vi "LSMcontroller_v58.vi"() -> ()   [LabVIEW 2015] (continued)
                n2596 = call <vilib>:"DAQmx Start Task.vi"("task/channels in"=w5606, "error in"=w5607) -> ("task out"=w5608:refnum<k21>, "error out"=w5609:errorcluster)  [unwired: 12 in]
                n2597 = call <vilib>:"DAQmx Stop Task.vi"("task/channels in"=w5608, "error in"=w5609) -> ("task out"=w5610:refnum<k21>, "error out"=w5611:errorcluster)  [unwired: 12 in]
                n2598 = call <vilib>:"DAQmx Clear Task.vi"("task in"=w5610, "error in"=w5611) -> ()  [unwired: 13 in, 1 out]
              }
            }
          }
          event "sealtest": Value Change {
            n2599 = event-data() -> ()  [unwired: 1 in, 6 out]
            n2600 = case shown="True" "sealtest" {
              frame False {
              }
              frame True {
                n2601 = stacked-sequence {
                  seq-local: [w5613 _ _ _ _ _] -> [_ w5646 _ w5698 _ _]
                  frame #0 {
                    n2602 = stacked-sequence {
                      tunnel: [_ w5625 _] -> w5613
                      frame #0 {
                        n2603 = call "2pparameters.vi"("command"="get") -> ("params out"=w5618:T12)  [unwired: 1 in]
                        n2604 = Unbundle By Name(w5618) -> ("autoshutter"=w5619:bool)
                        n2605 = local read "OCchecked?"() -> (w5616:bool)
                        n2606 = call "sealtestwfparams.vi"("command"="set") -> ()  [unwired: 6 in, 1 out]
                        n2607 = case shown="False" w5616 {
                          frame False {
                            n2608 = One Button Dialog(message="Is the OC gain correct?", button name ("OK")="ok") -> (true=w5620:bool)
                            n2609 = local write "OCchecked?"(w5620) -> ()
                          }
                          frame True {
                          }
                        }
                        n2610 = case shown="True" w5619 {
                          frame False {
                          }
                          frame True {
                            n2611 = call "shuttercontrol.vi"("command"="close") -> ()  [unwired: 1 in, 1 out]
                          }
                        }
                        n2612 = call "allAI-temp.vi"("command"=enum16{"get", "set", "clear", "append"}."clear") -> ()  [unwired: 3 in, 2 out]
                      }
                      frame #1 {
                        n2613 = call "sealtestwfparams.vi"("command"="get") -> ("Params out"=w5631:T25)  [unwired: 6 in]
                        n2614 = Unbundle By Name(w5631) -> ("AO parameters"=w5629:T1)
                        "AO parameters 2" <- w5629
                        n2615 = Index Array(array=w5629, index=0) -> (element=w5628:T26)
                        n2616 = call "generateRampedSquareWave_fromAOparameters.vi"("AO params"=w5628) -> ("Waveform"=w5624:waveform(dbl), "wflength"=w5625:i32)
                        "Waveform Graph" <- w5624
                        "wflength" <- w5625
                        n2617 = Build Array(w5624) -> (w5627:waveform(dbl)[])
                        n2618 = call "waveformssealtestbuffer.vi"("AO wf in"=w5627, "command"="set") -> ()  [unwired: 1 out]
                      }
                      frame #2 {
                        n2619 = local read "Vholding (mV)"() -> (w5634:sgl)
                        n2620 = local read "Current Clamp"() -> (w5640:bool)
                        n2621 = local read "Voltage Clamp"() -> (w5639:bool)
                        n2622 = local read "OCgain"() -> (w5635:sgl)
                        n2623 = local read "CC_ICgain"() -> (w5638:dbl)
                        n2624 = local read "holdon"() -> (w5633:bool)
                        n2625 = call "patchparameters.vi"("command"="get") -> ("Params out"=w5642:T15)  [unwired: 1 in]
                        n2626 = Bundle By Name(cluster=w5642, "VC"=w5639, "CC"=w5640, "CC_icg (pA/mv)"=w5638, "VC_icg (mV/mV)"=10.0, "OCG (mV/pA)"=w5635, "OVG (mV/mV)"=0.1, "Vhold (mV)"=w5634, "holdon"=w5633) -> (w5641:T15)
                        n2627 = call "patchparameters.vi"("Params in"=w5641, "command"="set") -> ()  [unwired: 1 out]
                      }
                    }
                  }
                  frame #1 {
                    w5645 = 2
                    n2628 = call "patchparameters.vi"("command"="get") -> ("Params out"=w5653:T15)  [unwired: 1 in]
                    n2629 = Unbundle By Name(w5653) -> ("holdon"=w5652:bool, "Vhold (mV)"=w5651:sgl, "CC_icg (pA/mv)"=w5659:sgl, "CC"=w5657:bool, "VC_icg (mV/mV)"=w5658:sgl)
                    n2630 = Select(t=w5659, s=w5657, f=w5658) -> (s? t:f=w5660:sgl)
                    n2631 = To Single Precision Float(number=0.001 ("y")) -> (single precision float=w5661:sgl)
                    n2632 = Compound Arithmetic op=MULTIPLY(w5651, w5660, w5661) -> (w5655:sgl)
                    n2633 = case shown="False" w5652 {
                      tunnel: w5655 -> [_ w5673]
                      tunnel: [0.0 w5673] -> w5648
                      frame False {
                      }
                      frame True {
                      }
                    }
                    n2634 = Greater Than 0?(x=w5645) -> (x > 0?=w5647:bool)
                    n2635 = case shown="True" w5647 {
                      tunnel: w5646 -> [_ w5662]
                      tunnel: w5645 -> [_ w5665]
                      frame False {
                      }
                      frame True {
                        n2636 = Initialize Array(sgl 0.0 ("element"), w5665, w5662) -> (w5663:sgl[][])
                        n2637 = call "allAI-temp.vi"("array in"=w5663, "command"=enum16{"get", "set", "clear", "append"}."set") -> ()  [unwired: 2 in, 2 out]
                      }
                    }
                    n2638 = flat-sequence {
                      tunnel: w5646 -> [w5669]
                      tunnel: w5646 -> [w5668]
                      tunnel: [w5668] -> w5650
                      tunnel: [w5667] -> w5649
                      tunnel: w5648 -> [w5667]
                      tunnel: w5650 -> [w5671]
                      tunnel: w5649 -> [w5670]
                      frame #0 {
                        n2639 = call "prepAI_sealtest.vi"("samples per channel"=w5669) -> ()  [unwired: 2 in]
                      }
                      frame #1 {
                        n2640 = call "prepAO_sealtest.vi"("Vhold"=w5670, "samples per channel"=w5671) -> ()  [unwired: 1 in]
                      }
                    }
                  }
                  frame #2 {
                    n2641 = stacked-sequence {
                      frame #0 {
                        n2642 = call "tempconfigAO.vi"("command"="get") -> ("Temp Config out"=w5677:T27)  [unwired: 1 in]
                        n2643 = Unbundle By Name(w5677) -> ("AO"=w5678:refnum<k21>[], "E_AO"=w5679:errorcluster[])
                        n2644 = for {
                          tunnel: w5678 -> [w5687] mode=indexing
                          tunnel: w5679 -> [w5686] mode=indexing
                          tunnel: [w5685] -> w5681 mode=indexing
                          tunnel: [w5684] -> w5682 mode=indexing
                          n2645 = call <vilib>:"DAQmx Start Task.vi"("task/channels in"=w5687, "error in"=w5686) -> ("task out"=w5685:refnum<k21>, "error out"=w5684:errorcluster)  [unwired: 12 in]
                        }
                        n2646 = call "tempconfigAO.vi"("command"="get") -> ("Temp Config out"=w5680:T27)  [unwired: 1 in]
                        n2647 = Bundle By Name(cluster=w5680, "AO"=w5681, "E_AO"=w5682) -> (w5683:T27)
                        n2648 = call "tempconfigAO.vi"("Temp Config in"=w5683, "command"="set") -> ()  [unwired: 1 out]
                      }
                      frame #1 {
                        n2649 = call "tempconfigAI.vi"("command"="get") -> ("Temp Config out"=w5689:T28)  [unwired: 1 in]
                        n2650 = Unbundle By Name(w5689) -> ("AI"=w5694:refnum<k21>, "E_AI"=w5695:errorcluster)
                        n2651 = call <vilib>:"DAQmx Start Task.vi"("task/channels in"=w5694, "error in"=w5695) -> ("task out"=w5696:refnum<k21>, "error out"=w5697:errorcluster)  [unwired: 12 in]
                        n2652 = call "tempconfigAI.vi"("command"="get") -> ("Temp Config out"=w5691:T28)  [unwired: 1 in]
                        n2653 = Bundle By Name(cluster=w5691, "AI"=w5696, "E_AI"=w5697) -> (w5693:T28)
                        n2654 = call "tempconfigAI.vi"("Temp Config in"=w5693, "command"="set") -> ()  [unwired: 1 out]
                      }
                    }
                  }
                  frame #3 {
                    n2655 = while {
                      tunnel: w5698 -> [w5699]
                      stop <- w5700 stop-if-true
                      n2656 = local read "sealtest"() -> (w5703:bool)
                      n2657 = Not(x=w5703) -> (.not. x?=w5702:bool)
                      n2658 = case shown="False" w5702 {
                        tunnel: w5699 -> [w5704 _]
                        frame False {
                          n2659 = stacked-sequence {
                            seq-local: [_ _ _ w5743 _ _] -> [_ _ _ _ w5799 _]
                            seq-local: [w5705 _ _ _ _ _] -> [_ w5714 _ w5736 w5788 w5819]
                            tunnel: w5704 -> [_ _ w5722 _ w5787 _]
                            frame #0 {
                              n2660 = call "patchparameters.vi"("command"="get") -> ("Params out"=w5712:T15)  [unwired: 1 in]
                              n2661 = local read "Vholding (mV)"() -> (w5709:sgl)
                              n2662 = Unbundle By Name(w5712) -> ("Vhold (mV)"=w5708:sgl, "holdon"=w5711:bool)
                              n2663 = local read "holdon"() -> (w5710:bool)
                              n2664 = Not Equal?(x=w5709, y=w5708) -> (x != y?=w5707:bool)
                              n2665 = Not Equal?(x=w5711, y=w5710) -> (x != y?=w5706:bool)
                              n2666 = Or(x=w5707, y=w5706) -> (x .or. y?=w5705:bool)
                            }
                            frame #1 {
                              n2667 = case shown="True" w5714 {
                                frame False {
                                }
                                frame True {
                                n2668 = local read "Vholding (mV)"() -> (w5717:sgl)
                                n2669 = local read "holdon"() -> (w5715:bool)
                                n2670 = call "patchparameters.vi"("command"="get") -> ("Params out"=w5718:T15)  [unwired: 1 in]
                                n2671 = Bundle By Name(cluster=w5718, "Vhold (mV)"=w5717, "holdon"=w5715) -> (w5716:T15)
                                n2672 = call "patchparameters.vi"("Params in"=w5716, "command"="set") -> ()  [unwired: 1 out]
                                }
                              }
                            }
                            frame #2 {
                              n2673 = call "tempconfigAI.vi"("command"="get") -> ("Temp Config out"=w5732:T28)  [unwired: 1 in]
                              n2674 = Unbundle By Name(w5732) -> ("AI"=w5731:refnum<k21>, "E_AI"=w5730:errorcluster)
                              n2675 = call-poly <vilib>:"DAQmx Read.vi"("task/channels in"=w5731, "number of samples per channel"=w5722, "timeout"=10.0, "error in"=w5730) -> ("task out"=w5726:refnum<k21>, "data"=w5723:i16[][], "error out"=w5735:errorcluster)  [unwired: 9 in]
                              n2676 = call "tempconfigAI.vi"("command"="get") -> ("Temp Config out"=w5727:T28)  [unwired: 1 in]
                              n2677 = Bundle By Name(cluster=w5727, "AI"=w5726, "E_AI"=w5735) -> (w5734:T28)
                              n2678 = To Single Precision Float(number=w5723) -> (single precision float=w5725:sgl[][])
                              n2679 = call "tempconfigAI.vi"("Temp Config in"=w5734, "command"="set") -> ()  [unwired: 1 out]
                              n2680 = call "allAI-temp.vi"("array in"=w5725, "command"=enum16{"get", "set", "clear", "append"}."set") -> ()  [unwired: 2 in, 2 out]
                            }
                            frame #3 {
                              n2681 = case shown="True" w5736 {
                                frame False {
                                }
                                frame True {
                                n2682 = call "tempconfigAO.vi"("command"="get") -> ("Temp Config out"=w5776:T27)  [unwired: 1 in]
                                n2683 = Unbundle By Name(w5776) -> ("AO"=w5775:refnum<k21>[], "E_AO"=w5774:errorcluster[])
                                n2684 = call "tempconfigAI.vi"("command"="get") -> ("Temp Config out"=w5763:T28)  [unwired: 1 in]
                                n2685 = Unbundle By Name(w5763) -> ("AI"=w5764:refnum<k21>, "E_AI"=w5765:errorcluster)
                                n2686 = for {
                                tunnel: w5775 -> [w5780] mode=indexing
                                tunnel: w5774 -> [w5779] mode=indexing
                                tunnel: [w5778] -> w5770 mode=indexing
                                n2687 = call <vilib>:"DAQmx Stop Task.vi"("task/channels in"=w5780, "error in"=w5779) -> ("task out"=w5781:refnum<k21>, "error out"=w5782:errorcluster)  [unwired: 12 in]
                                n2688 = call <vilib>:"DAQmx Clear Task.vi"("task in"=w5781, "error in"=w5782) -> ("error out"=w5778:errorcluster)  [unwired: 13 in]
                                }
                                n2689 = call <vilib>:"DAQmx Stop Task.vi"("task/channels in"=w5764, "error in"=w5765) -> ("task out"=w5761:refnum<k21>, "error out"=w5760:errorcluster)  [unwired: 12 in]
                                n2690 = call <vilib>:"DAQmx Clear Task.vi"("task in"=w5761, "error in"=w5760) -> ("error out"=w5759:errorcluster)  [unwired: 13 in]
                                n2691 = call "tempconfigAO.vi"("command"="get") -> ("Temp Config out"=w5771:T27)  [unwired: 1 in]
                                n2692 = Bundle By Name(cluster=w5771, "E_AO"=w5770) -> (w5769:T27)
                                n2693 = call "tempconfigAI.vi"("command"="get") -> ("Temp Config out"=w5767:T28)  [unwired: 1 in]
                                n2694 = Bundle By Name(cluster=w5767, "E_AI"=w5759) -> (w5758:T28)
                                n2695 = call "tempconfigAO.vi"("Temp Config in"=w5769, "command"="set") -> ()  [unwired: 1 out]
                                n2696 = call "tempconfigAI.vi"("Temp Config in"=w5758, "command"="set") -> ()  [unwired: 1 out]
                                }
                              }
                              n2697 = call "allAI-temp.vi"("command"=enum16{"get", "set", "clear", "append"}."get") -> ("array out"=w5740:sgl[][])  [unwired: 3 in, 1 out]
                              n2698 = call "tempconfigAI.vi"("command"="get") -> ("Temp Config out"=w5753:T28)  [unwired: 1 in]
                              n2699 = call "tempconfigAI.vi"("command"="get") -> ("Temp Config out"=w5755:T28)  [unwired: 1 in]
                              n2700 = Unbundle By Name(w5753) -> ("header"=w5751:dbl[])
                              n2701 = Unbundle By Name(w5755) -> ("header"=w5757:dbl[])
                              n2702 = Index Array(array=w5740, index (row) #1=1 ("index (row)"), index (row) #2=0 ("index (row)")) -> (element #1=w5738:sgl[], element #2=w5737:sgl[])  [unwired: 2 in]
                              n2703 = local read "OCgain"() -> (w5745:sgl)
                              n2704 = call "Unscaledtoscaled.vi"("Unscaled Data"=w5738, "Header Information"=w5751) -> ("Array"=w5750:sgl[])  [unwired: 1 in]
                              n2705 = call "Unscaledtoscaled.vi"("Unscaled Data"=w5737, "Header Information"=w5757) -> ("Array"=w5754:sgl[])  [unwired: 1 in]
                              n2706 = Multiply(x=w5750, y=0.1) -> (x*y=w5747:dbl[])
                              n2707 = Divide(x=w5754, y=w5745) -> (x/y=w5746:sgl[])
                              n2708 = Build Array(w5747, w5746) -> (w5749:dbl[][])
                              n2709 = Multiply(x=w5749, y=1000.0) -> (x*y=w5743:dbl[][])
                              "Patch readout" <- w5743
                            }
                            frame #4 {
                              n2710 = case shown="True" w5788 {
                                tunnel: w5787 -> [_ w5800]
                                frame False {
                                }
                                frame True {
                                n2711 = call "patchparameters.vi"("command"="get") -> ("Params out"=w5804:T15)  [unwired: 1 in]
                                n2712 = Unbundle By Name(w5804) -> ("holdon"=w5803:bool, "Vhold (mV)"=w5802:sgl, "CC_icg (pA/mv)"=w5810:sgl, "CC"=w5808:bool, "VC_icg (mV/mV)"=w5809:sgl)
                                n2713 = Select(t=w5810, s=w5808, f=w5809) -> (s? t:f=w5811:sgl)
                                n2714 = To Single Precision Float(number=0.001 ("y")) -> (single precision float=w5812:sgl)
                                n2715 = Compound Arithmetic op=MULTIPLY(w5802, w5811, w5812) -> (w5806:sgl)
                                n2716 = case shown="True" w5803 {
                                tunnel: w5806 -> [_ w5817]
                                tunnel: [0.0 w5817] -> w5801
                                frame False {
                                }
                                frame True {
                                }
                                }
                                n2717 = flat-sequence {
                                tunnel: w5800 -> [w5813]
                                tunnel: w5801 -> [w5815]
                                tunnel: w5800 -> [w5814]
                                frame #0 {
                                n2718 = call "prepAI_sealtest.vi"("samples per channel"=w5813) -> ()  [unwired: 2 in]
                                }
                                frame #1 {
                                n2719 = call "prepAO_sealtest.vi"("Vhold"=w5815, "samples per channel"=w5814) -> ()  [unwired: 1 in]
                                }
                                }
                                }
                              }
                              n2720 = call "sealtestwfparams.vi"("command"="get") -> ("Params out"=w5793:T25)  [unwired: 6 in]
                              n2721 = Unbundle By Name(w5793) -> ("AO parameters"=w5794:T1)
                              n2722 = Index Array(array=w5794, index=0) -> (element=w5796:T26)
                              n2723 = Unbundle By Name(w5796) -> ("Cycles"=w5791:dbl, "Start amplitude (V)"=w5790:dbl, "Sampling frequency (Hz)"=w5789:dbl)
                              n2724 = local read "fitpoints"() -> (w5797:dbl)
                              n2725 = script code="V=data(1,:);\nI=data(2,:);\ntres=mean(V);\nspc=(nsamp./ncyc);\nV=V(spc+1:end-spc);\nI=I(spc+1:end-spc);\ndV=mean(V(V>tres))-mean(V(V<tres))\nIcyc=reshape(I,[spc ncyc-2]);\nIcyc=Icyc';\nIcyc=mean(Icyc,1);\ndIss=mean(Icyc(floor(spc*0.15):floor(spc/2)-2))-mean(Icyc(spc*0.65:spc-2))\nRm=dV*1e3/dIss;\n[maxi,ind]=max(Icyc);\nIfit=Icyc(ind+1:ind+1+points-1)-0.5*(mean(Icyc(floor(spc*0.15):floor(spc/2)-2))+mean(Icyc(spc*0.65:spc-2)))\nt=(3:points-1+3)./srate*1000;\nt=t';\nIfit=Ifit';\nc=fit(t,Ifit, 'exp1');\ncoeffs=coeffvalues(c);\nIa=coeffs(1);\nRa=dV*1e3./Ia/2;\ntau=-1./coeffs(2);\ncap=tau/Ra*1000;"("data"=w5799, "nsamp"=w5787, "ncyc"=w5791, "maxV"=w5790, "points"=w5797, "srate"=w5789) -> ("cap"=w5786:dbl, "Ra"=w5785:dbl, "Icyc"=w5784:dbl[], "Rm"=w5783:dbl)  [unwired: 1 in, 1 out]
                              n2726 = local read "set as Rp?"() -> (w5798:bool)
                              n2727 = local write "Cmembrane"(w5786) -> ()
                              n2728 = local write "Rmembrane (MOhm)"(w5783) -> ()
                              n2729 = local write "Racces (MOhm)"(w5785) -> ()
                              n2730 = case shown="True" w5798 {
                                tunnel: w5783 -> [_ w5818]
                                frame False {
                                }
                                frame True {
                                n2731 = local write "Rpipette (MOhm)"(w5818) -> ()
                                }
                              }
                              n2732 = local write "Ifit"(w5784) -> ()
                            }
                            frame #5 {
                              n2733 = local read "set as Rp?"() -> (w5820:bool)
                              n2734 = case shown="True" w5819 {
                                frame False {
                                }
                                frame True {
                                n2735 = stacked-sequence {
                                frame #0 {
                                n2736 = call "tempconfigAO.vi"("command"="get") -> ("Temp Config out"=w5827:T27)  [unwired: 1 in]
                                n2737 = Unbundle By Name(w5827) -> ("AO"=w5826:refnum<k21>[], "E_AO"=w5825:errorcluster[])
                                n2738 = for {
                                tunnel: w5826 -> [w5834] mode=indexing
                                tunnel: w5825 -> [w5833] mode=indexing
                                tunnel: [w5832] -> w5823 mode=indexing
                                tunnel: [w5831] -> w5822 mode=indexing
                                n2739 = call <vilib>:"DAQmx Start Task.vi"("task/channels in"=w5834, "error in"=w5833) -> ("task out"=w5832:refnum<k21>, "error out"=w5831:errorcluster)  [unwired: 12 in]
                                }
                                n2740 = call "tempconfigAO.vi"("command"="get") -> ("Temp Config out"=w5824:T27)  [unwired: 1 in]
                                n2741 = Bundle By Name(cluster=w5824, "AO"=w5823, "E_AO"=w5822) -> (w5821:T27)
                                n2742 = call "tempconfigAO.vi"("Temp Config in"=w5821, "command"="set") -> ()  [unwired: 1 out]
                                }
                                frame #1 {
                                n2743 = call "tempconfigAI.vi"("command"="get") -> ("Temp Config out"=w5836:T28)  [unwired: 1 in]
                                n2744 = Unbundle By Name(w5836) -> ("AI"=w5841:refnum<k21>, "E_AI"=w5842:errorcluster)
                                n2745 = call <vilib>:"DAQmx Start Task.vi"("task/channels in"=w5841, "error in"=w5842) -> ("task out"=w5843:refnum<k21>, "error out"=w5844:errorcluster)  [unwired: 12 in]
                                n2746 = call "tempconfigAI.vi"("command"="get") -> ("Temp Config out"=w5838:T28)  [unwired: 1 in]
                                n2747 = Bundle By Name(cluster=w5838, "AI"=w5843, "E_AI"=w5844) -> (w5840:T28)
                                n2748 = call "tempconfigAI.vi"("Temp Config in"=w5840, "command"="set") -> ()  [unwired: 1 out]
                                }
                                }
                                }
                              }
                              n2749 = case shown="True" w5820 {
                                frame False {
                                }
                                frame True {
                                n2750 = local write "set as Rp?"(FALSE ("set as Rp?")) -> ()
                                }
                              }
                            }
                          }
                        }
                        frame True {
                        }
                      }
                      n2751 = local read "sealtest"() -> (w5701:bool)
                      n2752 = Not(x=w5701) -> (.not. x?=w5700:bool)
                    }
                  }
                  frame #4 {
                    n2753 = call "tempconfigAO.vi"("command"="get") -> ("Temp Config out"=w5871:T27)  [unwired: 1 in]
                    n2754 = Unbundle By Name(w5871) -> ("AO"=w5870:refnum<k21>[], "E_AO"=w5869:errorcluster[])
                    n2755 = call "configuration.vi"("command"="get") -> ("config out"=w5852:T13)  [unwired: 2 in, 1 out]
                    n2756 = call "tempconfigAI.vi"("command"="get") -> ("Temp Config out"=w5858:T28)  [unwired: 1 in]
                    n2757 = Unbundle By Name(w5852) -> ("Device 1 sampleclock out"=w5849:tag, "Device 1 Starttrigger out"=w5848:tag)
                    n2758 = Unbundle By Name(w5858) -> ("AI"=w5859:refnum<k21>, "E_AI"=w5860:errorcluster)
                    n2759 = for {
                      tunnel: w5870 -> [w5875] mode=indexing
                      tunnel: w5869 -> [w5874] mode=indexing
                      tunnel: [w5873] -> w5865 mode=indexing
                      n2760 = call <vilib>:"DAQmx Stop Task.vi"("task/channels in"=w5875, "error in"=w5874) -> ("task out"=w5876:refnum<k21>, "error out"=w5877:errorcluster)  [unwired: 12 in]
                      n2761 = call <vilib>:"DAQmx Clear Task.vi"("task in"=w5876, "error in"=w5877) -> ("error out"=w5873:errorcluster)  [unwired: 13 in]
                    }
                    n2762 = call <vilib>:"DAQmx Stop Task.vi"("task/channels in"=w5859, "error in"=w5860) -> ("task out"=w5856:refnum<k21>, "error out"=w5855:errorcluster)  [unwired: 12 in]
                    n2763 = call <vilib>:"DAQmx Disconnect Terminals.vi"("source terminal"=tag "/Dev1/ai/SampleClock", "destination terminal"=w5849) -> ("error out"=w5846:errorcluster)  [unwired: 13 in]
                    n2764 = call <vilib>:"DAQmx Clear Task.vi"("task in"=w5856, "error in"=w5855) -> ("error out"=w5854:errorcluster)  [unwired: 13 in]
                    n2765 = call "tempconfigAO.vi"("command"="get") -> ("Temp Config out"=w5866:T27)  [unwired: 1 in]
                    n2766 = Bundle By Name(cluster=w5866, "E_AO"=w5865) -> (w5864:T27)
                    n2767 = call "tempconfigAI.vi"("command"="get") -> ("Temp Config out"=w5862:T28)  [unwired: 1 in]
                    n2768 = Bundle By Name(cluster=w5862, "E_AI"=w5854) -> (w5853:T28)
                    n2769 = call "tempconfigAO.vi"("Temp Config in"=w5864, "command"="set") -> ()  [unwired: 1 out]
                    n2770 = call <vilib>:"DAQmx Disconnect Terminals.vi"("source terminal"=tag "/Dev1/ai/StartTrigger", "destination terminal"=w5848, "error in"=w5846) -> ()  [unwired: 12 in, 1 out]
                    n2771 = call "tempconfigAI.vi"("Temp Config in"=w5853, "command"="set") -> ()  [unwired: 1 out]
                  }
                  frame #5 {
                    w5880 = T23 4 items=["no dialog", "OK message", "continue or stop message", "OK message + warnings", "continue/stop + warnings"] ("type of dialog (OK msg:1)")
                    n2772 = call "displayerrors.vi"() -> ("error IO"=w5879:errorcluster)
                    n2773 = call "zeropatch.vi"() -> ()  [unwired: 12 in]
                    n2774 = call <vilib>:"Simple Error Handler.vi"("type of dialog (OK msg:1)"=w5880, "error in (no error)"=w5879) -> ("error out"=w5878:errorcluster)  [unwired: 3 in, 4 out]
                    n2775 = call <vilib>:"Clear Errors.vi"("error in (no error)"=w5878) -> ()  [unwired: 5 in, 2 out]
                  }
                }
              }
            }
          }
          event "readpatch": Value Change {
            n2776 = event-data() -> ()  [unwired: 1 in, 6 out]
            n2777 = local read "readpatch"() -> (w5881:bool)
            n2778 = case shown="True" w5881 {
              frame False {
              }
              frame True {
                n2779 = stacked-sequence {
                  seq-local: [w5882 _ _ _ _ _] -> [_ w5915 _ w5967 _ _]
                  frame #0 {
                    n2780 = stacked-sequence {
                      tunnel: [_ w5894 _] -> w5882
                      frame #0 {
                        n2781 = call "2pparameters.vi"("command"="get") -> ("params out"=w5887:T12)  [unwired: 1 in]
                        n2782 = Unbundle By Name(w5887) -> ("autoshutter"=w5888:bool)
                        n2783 = local read "OCchecked?"() -> (w5885:bool)
                        n2784 = call "sealtestwfparams.vi"("command"="set") -> ()  [unwired: 6 in, 1 out]
                        n2785 = case shown="False" w5885 {
                          frame False {
                            n2786 = One Button Dialog(message="Is the OC gain correct?", button name ("OK")="ok") -> (true=w5889:bool)
                            n2787 = local write "OCchecked?"(w5889) -> ()
                          }
                          frame True {
                          }
                        }
                        n2788 = case shown="True" w5888 {
                          frame False {
                          }
                          frame True {
                            n2789 = call "shuttercontrol.vi"("command"="close") -> ()  [unwired: 1 in, 1 out]
                          }
                        }
                        n2790 = call "allAI-temp.vi"("command"=enum16{"get", "set", "clear", "append"}."clear") -> ()  [unwired: 3 in, 2 out]
                      }
                      frame #1 {
                        n2791 = call "sealtestwfparams.vi"("command"="get") -> ("Params out"=w5900:T25)  [unwired: 6 in]
                        n2792 = Unbundle By Name(w5900) -> ("AO parameters"=w5898:T1)
                        n2793 = Index Array(array=w5898, index=1) -> (element=w5897:T26)
                        n2794 = call "generateRampedSquareWave_fromAOparameters.vi"("AO params"=w5897) -> ("Waveform"=w5893:waveform(dbl), "wflength"=w5894:i32)
                        n2795 = Build Array(w5893) -> (w5896:waveform(dbl)[])
                        n2796 = call "waveformssealtestbuffer.vi"("AO wf in"=w5896, "command"="set") -> ()  [unwired: 1 out]
                      }
                      frame #2 {
                        n2797 = local read "Vholding (mV)"() -> (w5903:sgl)
                        n2798 = local read "Current Clamp"() -> (w5909:bool)
                        n2799 = local read "Voltage Clamp"() -> (w5908:bool)
                        n2800 = local read "OCgain"() -> (w5904:sgl)
                        n2801 = local read "CC_ICgain"() -> (w5907:dbl)
                        n2802 = local read "holdon"() -> (w5902:bool)
                        n2803 = call "patchparameters.vi"("command"="get") -> ("Params out"=w5911:T15)  [unwired: 1 in]
                        n2804 = Bundle By Name(cluster=w5911, "VC"=w5908, "CC"=w5909, "CC_icg (pA/mv)"=w5907, "VC_icg (mV/mV)"=10.0, "OCG (mV/pA)"=w5904, "OVG (mV/mV)"=0.1, "Vhold (mV)"=w5903, "holdon"=w5902) -> (w5910:T15)
                        n2805 = call "patchparameters.vi"("Params in"=w5910, "command"="set") -> ()  [unwired: 1 out]
                      }
                    }
                  }
                  frame #1 {
                    w5914 = 2
                    n2806 = call "patchparameters.vi"("command"="get") -> ("Params out"=w5922:T15)  [unwired: 1 in]
                    n2807 = Unbundle By Name(w5922) -> ("holdon"=w5921:bool, "Vhold (mV)"=w5920:sgl, "CC_icg (pA/mv)"=w5928:sgl, "CC"=w5926:bool, "VC_icg (mV/mV)"=w5927:sgl)
                    n2808 = Select(t=w5928, s=w5926, f=w5927) -> (s? t:f=w5929:sgl)
                    n2809 = To Single Precision Float(number=0.001 ("y")) -> (single precision float=w5930:sgl)
                    n2810 = Compound Arithmetic op=MULTIPLY(w5920, w5929, w5930) -> (w5924:sgl)
                    n2811 = case shown="False" w5921 {
                      tunnel: w5924 -> [_ w5942]
                      tunnel: [0.0 w5942] -> w5917
                      frame False {
                      }
                      frame True {
                      }
                    }
                    n2812 = Greater Than 0?(x=w5914) -> (x > 0?=w5916:bool)
                    n2813 = case shown="True" w5916 {
                      tunnel: w5915 -> [_ w5931]
                      tunnel: w5914 -> [_ w5934]
                      frame False {
                      }
                      frame True {
                        n2814 = Initialize Array(sgl 0.0 ("element"), w5934, w5931) -> (w5932:sgl[][])
                        n2815 = call "allAI-temp.vi"("array in"=w5932, "command"=enum16{"get", "set", "clear", "append"}."set") -> ()  [unwired: 2 in, 2 out]
                      }
                    }
                    n2816 = flat-sequence {
                      tunnel: w5915 -> [w5938]
                      tunnel: w5915 -> [w5937]
                      tunnel: [w5937] -> w5919
                      tunnel: [w5936] -> w5918
                      tunnel: w5917 -> [w5936]
                      tunnel: w5919 -> [w5940]
                      tunnel: w5918 -> [w5939]
                      frame #0 {
                        n2817 = call "prepAI_sealtest.vi"("samples per channel"=w5938) -> ()  [unwired: 2 in]
                      }
                      frame #1 {
                        n2818 = call "prepAO_sealtest.vi"("Vhold"=w5939, "samples per channel"=w5940) -> ()  [unwired: 1 in]
                      }
                    }
                  }
                  frame #2 {
                    n2819 = stacked-sequence {
                      frame #0 {
                        n2820 = call "tempconfigAO.vi"("command"="get") -> ("Temp Config out"=w5946:T27)  [unwired: 1 in]
                        n2821 = Unbundle By Name(w5946) -> ("AO"=w5947:refnum<k21>[], "E_AO"=w5948:errorcluster[])
                        n2822 = for {
                          tunnel: w5947 -> [w5956] mode=indexing
                          tunnel: w5948 -> [w5955] mode=indexing
                          tunnel: [w5954] -> w5950 mode=indexing
                          tunnel: [w5953] -> w5951 mode=indexing
                          n2823 = call <vilib>:"DAQmx Start Task.vi"("task/channels in"=w5956, "error in"=w5955) -> ("task out"=w5954:refnum<k21>, "error out"=w5953:errorcluster)  [unwired: 12 in]
                        }
                        n2824 = call "tempconfigAO.vi"("command"="get") -> ("Temp Config out"=w5949:T27)  [unwired: 1 in]
                        n2825 = Bundle By Name(cluster=w5949, "AO"=w5950, "E_AO"=w5951) -> (w5952:T27)
                        n2826 = call "tempconfigAO.vi"("Temp Config in"=w5952, "command"="set") -> ()  [unwired: 1 out]
                      }
                      frame #1 {
                        n2827 = call "tempconfigAI.vi"("command"="get") -> ("Temp Config out"=w5958:T28)  [unwired: 1 in]
                        n2828 = Unbundle By Name(w5958) -> ("AI"=w5963:refnum<k21>, "E_AI"=w5964:errorcluster)
                        n2829 = call <vilib>:"DAQmx Start Task.vi"("task/channels in"=w5963, "error in"=w5964) -> ("task out"=w5965:refnum<k21>, "error out"=w5966:errorcluster)  [unwired: 12 in]
                        n2830 = call "tempconfigAI.vi"("command"="get") -> ("Temp Config out"=w5960:T28)  [unwired: 1 in]
                        n2831 = Bundle By Name(cluster=w5960, "AI"=w5965, "E_AI"=w5966) -> (w5962:T28)
                        n2832 = call "tempconfigAI.vi"("Temp Config in"=w5962, "command"="set") -> ()  [unwired: 1 out]
                      }
                    }
                  }
                  frame #3 {
                    n2833 = while {
                      tunnel: w5967 -> [w5968]
                      stop <- w5969 stop-if-true
                      n2834 = local read "readpatch"() -> (w5972:bool)
                      n2835 = Not(x=w5972) -> (.not. x?=w5971:bool)
                      n2836 = case shown="True" w5971 {
                        tunnel: w5968 -> [w5973 _]
                        frame False {
                          n2837 = stacked-sequence {
                            seq-local: [w5974 _ _ _ _ _] -> [_ w5983 _ w6006 w6053 w6072]
                            tunnel: w5973 -> [_ _ w5991 _ w6052 _]
                            frame #0 {
                              n2838 = call "patchparameters.vi"("command"="get") -> ("Params out"=w5981:T15)  [unwired: 1 in]
                              n2839 = local read "Vholding (mV)"() -> (w5978:sgl)
                              n2840 = Unbundle By Name(w5981) -> ("Vhold (mV)"=w5977:sgl, "holdon"=w5980:bool)
                              n2841 = local read "holdon"() -> (w5979:bool)
                              n2842 = Not Equal?(x=w5978, y=w5977) -> (x != y?=w5976:bool)
                              n2843 = Not Equal?(x=w5980, y=w5979) -> (x != y?=w5975:bool)
                              n2844 = Or(x=w5976, y=w5975) -> (x .or. y?=w5974:bool)
                            }
                            frame #1 {
                              n2845 = case shown="False" w5983 {
                                frame False {
                                }
                                frame True {
                                n2846 = local read "Vholding (mV)"() -> (w5986:sgl)
                                n2847 = local read "holdon"() -> (w5984:bool)
                                n2848 = call "patchparameters.vi"("command"="get") -> ("Params out"=w5987:T15)  [unwired: 1 in]
                                n2849 = Bundle By Name(cluster=w5987, "Vhold (mV)"=w5986, "holdon"=w5984) -> (w5985:T15)
                                n2850 = call "patchparameters.vi"("Params in"=w5985, "command"="set") -> ()  [unwired: 1 out]
                                }
                              }
                            }
                            frame #2 {
                              n2851 = call "tempconfigAI.vi"("command"="get") -> ("Temp Config out"=w6001:T28)  [unwired: 1 in]
                              n2852 = Unbundle By Name(w6001) -> ("AI"=w6000:refnum<k21>, "E_AI"=w5999:errorcluster)
                              n2853 = call-poly <vilib>:"DAQmx Read.vi"("task/channels in"=w6000, "number of samples per channel"=w5991, "timeout"=10.0, "error in"=w5999) -> ("task out"=w5995:refnum<k21>, "data"=w5992:i16[][], "error out"=w6004:errorcluster)  [unwired: 9 in]
                              n2854 = call "tempconfigAI.vi"("command"="get") -> ("Temp Config out"=w5996:T28)  [unwired: 1 in]
                              n2855 = Bundle By Name(cluster=w5996, "AI"=w5995, "E_AI"=w6004) -> (w6003:T28)
                              n2856 = To Single Precision Float(number=w5992) -> (single precision float=w5994:sgl[][])
                              n2857 = call "tempconfigAI.vi"("Temp Config in"=w6003, "command"="set") -> ()  [unwired: 1 out]
                              n2858 = call "allAI-temp.vi"("array in"=w5994, "command"=enum16{"get", "set", "clear", "append"}."set") -> ()  [unwired: 2 in, 2 out]
                            }
                            frame #3 {
                              n2859 = case shown="True" w6006 {
                                frame False {
                                }
                                frame True {
                                n2860 = call "tempconfigAO.vi"("command"="get") -> ("Temp Config out"=w6045:T27)  [unwired: 1 in]
                                n2861 = Unbundle By Name(w6045) -> ("AO"=w6044:refnum<k21>[], "E_AO"=w6043:errorcluster[])
                                n2862 = call "tempconfigAI.vi"("command"="get") -> ("Temp Config out"=w6032:T28)  [unwired: 1 in]
                                n2863 = Unbundle By Name(w6032) -> ("AI"=w6033:refnum<k21>, "E_AI"=w6034:errorcluster)
                                n2864 = for {
                                tunnel: w6044 -> [w6049] mode=indexing
                                tunnel: w6043 -> [w6048] mode=indexing
                                tunnel: [w6047] -> w6039 mode=indexing
                                n2865 = call <vilib>:"DAQmx Stop Task.vi"("task/channels in"=w6049, "error in"=w6048) -> ("task out"=w6050:refnum<k21>, "error out"=w6051:errorcluster)  [unwired: 12 in]
                                n2866 = call <vilib>:"DAQmx Clear Task.vi"("task in"=w6050, "error in"=w6051) -> ("error out"=w6047:errorcluster)  [unwired: 13 in]
                                }
                                n2867 = call <vilib>:"DAQmx Stop Task.vi"("task/channels in"=w6033, "error in"=w6034) -> ("task out"=w6030:refnum<k21>, "error out"=w6029:errorcluster)  [unwired: 12 in]
                                n2868 = call <vilib>:"DAQmx Clear Task.vi"("task in"=w6030, "error in"=w6029) -> ("error out"=w6028:errorcluster)  [unwired: 13 in]
                                n2869 = call "tempconfigAO.vi"("command"="get") -> ("Temp Config out"=w6040:T27)  [unwired: 1 in]
                                n2870 = Bundle By Name(cluster=w6040, "E_AO"=w6039) -> (w6038:T27)
                                n2871 = call "tempconfigAI.vi"("command"="get") -> ("Temp Config out"=w6036:T28)  [unwired: 1 in]
                                n2872 = Bundle By Name(cluster=w6036, "E_AI"=w6028) -> (w6027:T28)
                                n2873 = call "tempconfigAO.vi"("Temp Config in"=w6038, "command"="set") -> ()  [unwired: 1 out]
                                n2874 = call "tempconfigAI.vi"("Temp Config in"=w6027, "command"="set") -> ()  [unwired: 1 out]
                                }
                              }
                              n2875 = call "allAI-temp.vi"("command"=enum16{"get", "set", "clear", "append"}."get") -> ("array out"=w6010:sgl[][])  [unwired: 3 in, 1 out]
                              n2876 = call "tempconfigAI.vi"("command"="get") -> ("Temp Config out"=w6022:T28)  [unwired: 1 in]
                              n2877 = call "tempconfigAI.vi"("command"="get") -> ("Temp Config out"=w6024:T28)  [unwired: 1 in]
                              n2878 = Unbundle By Name(w6022) -> ("header"=w6020:dbl[])
                              n2879 = Unbundle By Name(w6024) -> ("header"=w6026:dbl[])
                              n2880 = Index Array(array=w6010, index (row) #1=1 ("index (row)"), index (row) #2=0 ("index (row)")) -> (element #1=w6008:sgl[], element #2=w6007:sgl[])  [unwired: 2 in]
                              n2881 = local read "OCgain"() -> (w6014:sgl)
                              n2882 = call "Unscaledtoscaled.vi"("Unscaled Data"=w6008, "Header Information"=w6020) -> ("Array"=w6019:sgl[])  [unwired: 1 in]
                              n2883 = call "Unscaledtoscaled.vi"("Unscaled Data"=w6007, "Header Information"=w6026) -> ("Array"=w6023:sgl[])  [unwired: 1 in]
                              n2884 = Multiply(x=w6019, y=0.1) -> (x*y=w6016:dbl[])
                              n2885 = Divide(x=w6023, y=w6014) -> (x/y=w6015:sgl[])
                              n2886 = Build Array(w6016, w6015) -> (w6018:dbl[][])
                              n2887 = Multiply(x=w6018, y=1000.0) -> (x*y=w6005:dbl[][])
                              n2888 = local write "Patch readout"(w6005) -> ()
                            }
                            frame #4 {
                              n2889 = case shown="True" w6053 {
                                tunnel: w6052 -> [_ w6054]
                                frame False {
                                }
                                frame True {
                                n2890 = call "patchparameters.vi"("command"="get") -> ("Params out"=w6058:T15)  [unwired: 1 in]
                                n2891 = Unbundle By Name(w6058) -> ("holdon"=w6057:bool, "Vhold (mV)"=w6056:sgl, "CC_icg (pA/mv)"=w6064:sgl, "CC"=w6062:bool, "VC_icg (mV/mV)"=w6063:sgl)
                                n2892 = Select(t=w6064, s=w6062, f=w6063) -> (s? t:f=w6065:sgl)
                                n2893 = To Single Precision Float(number=0.001 ("y")) -> (single precision float=w6066:sgl)
                                n2894 = Compound Arithmetic op=MULTIPLY(w6056, w6065, w6066) -> (w6060:sgl)
                                n2895 = case shown="True" w6057 {
                                tunnel: w6060 -> [_ w6071]
                                tunnel: [0.0 w6071] -> w6055
                                frame False {
                                }
                                frame True {
                                }
                                }
                                n2896 = flat-sequence {
                                tunnel: w6054 -> [w6067]
                                tunnel: w6055 -> [w6069]
                                tunnel: w6054 -> [w6068]
                                frame #0 {
                                n2897 = call "prepAI_sealtest.vi"("samples per channel"=w6067) -> ()  [unwired: 2 in]
                                }
                                frame #1 {
                                n2898 = call "prepAO_sealtest.vi"("Vhold"=w6069, "samples per channel"=w6068) -> ()  [unwired: 1 in]
                                }
                                }
                                }
                              }
                            }
                            frame #5 {
                              n2899 = case shown="True" w6072 {
                                frame False {
                                }
                                frame True {
                                n2900 = stacked-sequence {
                                frame #0 {
                                n2901 = call "tempconfigAO.vi"("command"="get") -> ("Temp Config out"=w6079:T27)  [unwired: 1 in]
                                n2902 = Unbundle By Name(w6079) -> ("AO"=w6078:refnum<k21>[], "E_AO"=w6077:errorcluster[])
                                n2903 = for {
                                tunnel: w6078 -> [w6086] mode=indexing
                                tunnel: w6077 -> [w6085] mode=indexing
                                tunnel: [w6084] -> w6075 mode=indexing
                                tunnel: [w6083] -> w6074 mode=indexing
                                n2904 = call <vilib>:"DAQmx Start Task.vi"("task/channels in"=w6086, "error in"=w6085) -> ("task out"=w6084:refnum<k21>, "error out"=w6083:errorcluster)  [unwired: 12 in]
                                }
                                n2905 = call "tempconfigAO.vi"("command"="get") -> ("Temp Config out"=w6076:T27)  [unwired: 1 in]
                                n2906 = Bundle By Name(cluster=w6076, "AO"=w6075, "E_AO"=w6074) -> (w6073:T27)
                                n2907 = call "tempconfigAO.vi"("Temp Config in"=w6073, "command"="set") -> ()  [unwired: 1 out]
                                }
                                frame #1 {
                                n2908 = call "tempconfigAI.vi"("command"="get") -> ("Temp Config out"=w6088:T28)  [unwired: 1 in]
                                n2909 = Unbundle By Name(w6088) -> ("AI"=w6093:refnum<k21>, "E_AI"=w6094:errorcluster)
                                n2910 = call <vilib>:"DAQmx Start Task.vi"("task/channels in"=w6093, "error in"=w6094) -> ("task out"=w6095:refnum<k21>, "error out"=w6096:errorcluster)  [unwired: 12 in]
                                n2911 = call "tempconfigAI.vi"("command"="get") -> ("Temp Config out"=w6090:T28)  [unwired: 1 in]
                                n2912 = Bundle By Name(cluster=w6090, "AI"=w6095, "E_AI"=w6096) -> (w6092:T28)
                                n2913 = call "tempconfigAI.vi"("Temp Config in"=w6092, "command"="set") -> ()  [unwired: 1 out]
                                }
                                }
                                }
                              }
                            }
                          }
                        }
                        frame True {
                        }
                      }
                      n2914 = local read "readpatch"() -> (w5970:bool)
                      n2915 = Not(x=w5970) -> (.not. x?=w5969:bool)
                    }
                  }
                  frame #4 {
                    n2916 = call "tempconfigAO.vi"("command"="get") -> ("Temp Config out"=w6122:T27)  [unwired: 1 in]
                    n2917 = Unbundle By Name(w6122) -> ("AO"=w6121:refnum<k21>[], "E_AO"=w6120:errorcluster[])
                    n2918 = call "configuration.vi"("command"="get") -> ("config out"=w6103:T13)  [unwired: 2 in, 1 out]
                    n2919 = call "tempconfigAI.vi"("command"="get") -> ("Temp Config out"=w6109:T28)  [unwired: 1 in]
                    n2920 = Unbundle By Name(w6103) -> ("Device 1 sampleclock out"=w6100:tag, "Device 1 Starttrigger out"=w6099:tag)
                    n2921 = Unbundle By Name(w6109) -> ("AI"=w6110:refnum<k21>, "E_AI"=w6111:errorcluster)
                    n2922 = for {
                      tunnel: w6121 -> [w6126] mode=indexing
                      tunnel: w6120 -> [w6125] mode=indexing
                      tunnel: [w6124] -> w6116 mode=indexing
                      n2923 = call <vilib>:"DAQmx Stop Task.vi"("task/channels in"=w6126, "error in"=w6125) -> ("task out"=w6127:refnum<k21>, "error out"=w6128:errorcluster)  [unwired: 12 in]
                      n2924 = call <vilib>:"DAQmx Clear Task.vi"("task in"=w6127, "error in"=w6128) -> ("error out"=w6124:errorcluster)  [unwired: 13 in]
                    }
                    n2925 = call <vilib>:"DAQmx Stop Task.vi"("task/channels in"=w6110, "error in"=w6111) -> ("task out"=w6107:refnum<k21>, "error out"=w6106:errorcluster)  [unwired: 12 in]
                    n2926 = call <vilib>:"DAQmx Disconnect Terminals.vi"("source terminal"=tag "/Dev1/ai/SampleClock", "destination terminal"=w6100) -> ("error out"=w6097:errorcluster)  [unwired: 13 in]
                    n2927 = call <vilib>:"DAQmx Clear Task.vi"("task in"=w6107, "error in"=w6106) -> ("error out"=w6105:errorcluster)  [unwired: 13 in]
                    n2928 = call "tempconfigAO.vi"("command"="get") -> ("Temp Config out"=w6117:T27)  [unwired: 1 in]
                    n2929 = Bundle By Name(cluster=w6117, "E_AO"=w6116) -> (w6115:T27)
                    n2930 = call "tempconfigAI.vi"("command"="get") -> ("Temp Config out"=w6113:T28)  [unwired: 1 in]
                    n2931 = Bundle By Name(cluster=w6113, "E_AI"=w6105) -> (w6104:T28)
                    n2932 = call "tempconfigAO.vi"("Temp Config in"=w6115, "command"="set") -> ()  [unwired: 1 out]
                    n2933 = call <vilib>:"DAQmx Disconnect Terminals.vi"("source terminal"=tag "/Dev1/ai/StartTrigger", "destination terminal"=w6099, "error in"=w6097) -> ()  [unwired: 12 in, 1 out]
                    n2934 = call "tempconfigAI.vi"("Temp Config in"=w6104, "command"="set") -> ()  [unwired: 1 out]
                  }
                  frame #5 {
                    w6131 = T23 4 items=["no dialog", "OK message", "continue or stop message", "OK message + warnings", "continue/stop + warnings"] ("type of dialog (OK msg:1)")
                    n2935 = call "displayerrors.vi"() -> ("error IO"=w6130:errorcluster)
                    n2936 = call "zeropatch.vi"() -> ()  [unwired: 12 in]
                    n2937 = call <vilib>:"Simple Error Handler.vi"("type of dialog (OK msg:1)"=w6131, "error in (no error)"=w6130) -> ("error out"=w6129:errorcluster)  [unwired: 3 in, 4 out]
                    n2938 = call <vilib>:"Clear Errors.vi"("error in (no error)"=w6129) -> ()  [unwired: 5 in, 2 out]
                  }
                }
              }
            }
          }
          event "Current Clamp": Value Change {
            n2939 = event-data() -> ()  [unwired: 1 in, 6 out]
            n2940 = local read "Current Clamp"() -> (w6136:bool)
            n2941 = property on="Vholding (mV)" class="DigNum (strict)"("Caption.Text"="Ihold (pA)") -> ()  [unwired: 2 in, 2 out]
            n2942 = Not(x=w6136) -> (.not. x?=w6135:bool)
            n2943 = property on="Voltage Clamp" class="Bool (strict)"("Value"=w6135) -> ()  [unwired: 2 in, 2 out]
            n2944 = One Button Dialog(message="Have you switched the HEKA to CC and changed the external input cable?", button name ("OK")="Ok") -> ()  [unwired: 1 out]
          }
          event "Voltage Clamp": Value Change {
            n2945 = event-data() -> ()  [unwired: 1 in, 6 out]
            n2946 = local read "Voltage Clamp"() -> (w6141:bool)
            n2947 = Not(x=w6141) -> (.not. x?=w6140:bool)
            n2948 = property on="Current Clamp" class="Bool (strict)"("Value"=w6140) -> ()  [unwired: 2 in, 2 out]
            n2949 = One Button Dialog(message="Have you switched the HEKA to VC and changed the external input cable?", button name ("OK")="Ok") -> ()  [unwired: 1 out]
            n2950 = property on="Vholding (mV)" class="DigNum (strict)"("Caption.Text"="Vhold (mV)") -> ()  [unwired: 2 in, 2 out]
          }
          event "OCgain": Value Change {
            n2951 = event-data() -> ()  [unwired: 1 in, 6 out]
            n2952 = local read "OCgain"() -> (w6144:sgl)
            n2953 = Less?(x=w6144, y=0.3) -> (x < y?=w6142:bool)
            n2954 = case shown="True" w6142 {
              frame False {
                w6145 = 10.0 items=["0.1"=10.0, "10"=0.1] ("CC_ICgain")
                n2955 = local write "CC_ICgain"(w6145) -> ()
              }
              frame True {
                w6146 = 0.1 items=["0.1"=10.0, "10"=0.1] ("CC_ICgain")
                n2956 = local write "CC_ICgain"(w6146) -> ()
              }
            }
          }
          event "holdon": Value Change {
            n2957 = event-data() -> ()  [unwired: 1 in, 6 out]
            n2958 = stacked-sequence {
              frame #0 {
                n2959 = local read "Vholding (mV)"() -> (w6150:sgl)
                n2960 = local read "holdon"() -> (w6147:bool)
                n2961 = call "patchparameters.vi"("command"="get") -> ("Params out"=w6151:T15)  [unwired: 1 in]
                n2962 = Bundle By Name(cluster=w6151, "Vhold (mV)"=w6150, "holdon"=w6147) -> (w6148:T15)
                n2963 = call "patchparameters.vi"("Params in"=w6148, "command"="set") -> ()  [unwired: 1 out]
              }
              frame #1 {
                n2964 = call "zeropatch.vi"() -> ()  [unwired: 12 in]
              }
            }
          }
          event "Vholding (mV)": Value Change {
            n2965 = event-data() -> ()  [unwired: 1 in, 6 out]
            n2966 = local read "holdon"() -> (w6153:bool)
            n2967 = case shown="True" w6153 {
              frame False {
              }
              frame True {
                n2968 = stacked-sequence {
                  frame #0 {
                    n2969 = local read "Vholding (mV)"() -> (w6156:sgl)
                    n2970 = local read "holdon"() -> (w6157:bool)
                    n2971 = call "patchparameters.vi"("command"="get") -> ("Params out"=w6158:T15)  [unwired: 1 in]
                    n2972 = Bundle By Name(cluster=w6158, "Vhold (mV)"=w6156, "holdon"=w6157) -> (w6154:T15)
                    n2973 = call "patchparameters.vi"("Params in"=w6154, "command"="set") -> ()  [unwired: 1 out]
                  }
                  frame #1 {
                    n2974 = call "zeropatch.vi"() -> ()  [unwired: 12 in]
                  }
                }
              }
            }
          }
          event "AI channels": Value Change {
            n2975 = event-data() -> ()  [unwired: 1 in, 6 out]
            n2976 = local read "CI channels"() -> (w6167:i32[])
            n2977 = local read "AI channels"() -> (w6168:i32[])
            n2978 = call "configuration.vi"("command"="get") -> ("config out"=w6161:T13)  [unwired: 2 in, 1 out]
            n2979 = Unbundle By Name(w6161) -> ("CI names"=w6162:string[], "AI names"=w6163:string[])
            n2980 = for {
              tunnel: w6167 -> [w6173] mode=indexing
              tunnel: w6162 -> [w6174]
              tunnel: [w6172] -> w6164 mode=indexing
              n2981 = Index Array(array=w6174, index=w6173) -> (element=w6172:string)
            }
            n2982 = for {
              tunnel: w6168 -> [w6170] mode=indexing
              tunnel: w6163 -> [w6171]
              tunnel: [w6169] -> w6165 mode=indexing
              n2983 = Index Array(array=w6171, index=w6170) -> (element=w6169:string)
            }
            n2984 = Build Array (concatenate)(w6164, w6165) -> (w6166:string[])
            n2985 = property on="image1list" class="Ring (strict)"("Strings []"=w6166) -> ()  [unwired: 2 in, 2 out]
            n2986 = property on="image2list" class="Ring (strict)"("Strings []"=w6166) -> ()  [unwired: 2 in, 2 out]
          }
          event "CI channels": Value Change {
            n2987 = event-data() -> ()  [unwired: 1 in, 6 out]
            n2988 = local read "CI channels"() -> (w6182:i32[])
            n2989 = local read "AI channels"() -> (w6183:i32[])
            n2990 = call "configuration.vi"("command"="get") -> ("config out"=w6176:T13)  [unwired: 2 in, 1 out]
            n2991 = Unbundle By Name(w6176) -> ("CI names"=w6177:string[], "AI names"=w6178:string[])
            n2992 = for {
              tunnel: w6182 -> [w6188] mode=indexing
              tunnel: w6177 -> [w6189]
              tunnel: [w6187] -> w6179 mode=indexing
              n2993 = Index Array(array=w6189, index=w6188) -> (element=w6187:string)
            }
            n2994 = for {
              tunnel: w6183 -> [w6185] mode=indexing
              tunnel: w6178 -> [w6186]
              tunnel: [w6184] -> w6180 mode=indexing
              n2995 = Index Array(array=w6186, index=w6185) -> (element=w6184:string)
            }
            n2996 = Build Array (concatenate)(w6179, w6180) -> (w6181:string[])
            n2997 = property on="image1list" class="Ring (strict)"("Strings []"=w6181) -> ()  [unwired: 2 in, 2 out]
            n2998 = property on="image2list" class="Ring (strict)"("Strings []"=w6181) -> ()  [unwired: 2 in, 2 out]
          }
          event "setdatdir": Value Change {
            n2999 = event-data() -> ()  [unwired: 1 in, 5 out]
            n3000 = case shown="True" "setdatdir" {
              frame False {
              }
              frame True {
                n3001 = stacked-sequence {
                  frame #0 {
                    n3002 = local read "data dir"() -> (w6191:path)
                    n3003 = call "File Dialog"("start path"=w6191, "prompt"="Please select data directory...") -> ("selected path"=w6193:path, "cancelled"=w6192:bool, "error out"=w6194:errorcluster)  [unwired: 10 in, 1 out]
                    n3004 = case shown="False" w6192 {
                      tunnel: w6193 -> [w6202 _]
                      tunnel: w6194 -> [w6199 w6205]
                      tunnel: [w6197 w6205] -> w6196
                      frame False {
                        n3005 = local write "data dir"(w6202) -> ()
                        n3006 = call "configuration.vi"("error in"=w6199, "command"="get") -> ("Error out"=w6198:errorcluster, "config out"=w6204:T13)  [unwired: 1 in]
                        n3007 = Bundle By Name(cluster=w6204, "master data dir"=w6202) -> (w6203:T13)
                        n3008 = call "configuration.vi"("error in"=w6198, "config in"=w6203, "command"="set") -> ("Error out"=w6197:errorcluster)  [unwired: 1 out]
                      }
                      frame True {
                      }
                    }
                    n3009 = local write "status"(w6196) -> ()
                  }
                  frame #1 {
                    n3010 = property on="setdatdir" class="Bool (strict)"("Value"=FALSE ("setdatdir")) -> ()  [unwired: 2 in, 2 out]
                  }
                }
              }
            }
          }
          event "Shutter": Value Change {
            n3011 = event-data() -> ()  [unwired: 1 in, 5 out]
            n3012 = case shown="False" "Shutter" {
              frame False {
                n3013 = call "shuttercontrol.vi"("command"="close") -> ()  [unwired: 1 in, 1 out]
              }
              frame True {
                n3014 = call "shuttercontrol.vi"("command"="open") -> ()  [unwired: 1 in, 1 out]
              }
            }
          }
          event "ROI": Value Change {
            n3015 = event-data() -> ()  [unwired: 1 in, 5 out]
            n3016 = local read "ROI"() -> (w6210:bool)
            n3017 = case shown="True" w6210 {
              frame False {
              }
              frame True {
                n3018 = stacked-sequence {
                  frame #0 {
                    n3019 = local read "Square pixels"() -> (w6227:bool)
                    n3020 = local read "square matrix"() -> (w6226:bool)
                    n3021 = local read "Vx-max ref"() -> (w6232:dbl)
                    n3022 = local read "Vx-min ref"() -> (w6231:dbl)
                    n3023 = local read "Vy-min ref"() -> (w6228:dbl)
                    n3024 = local read "ypixels ref"() -> (w6230:i32)
                    n3025 = local read "Vy-max ref"() -> (w6229:dbl)
                    n3026 = local read "xpixels ref"() -> (w6233:i32)
                    n3027 = local read "Angle ref"() -> (w6225:dbl)
                    n3028 = local read "Colormap"() -> (w6234:i32)
                    n3029 = call "2pparameters.vi"("command"="get") -> ("params out"=w6237:T12)  [unwired: 1 in]
                    n3030 = Bundle By Name(cluster=w6237, "Xpixels Img"=w6233, "Vx-min Img"=w6231, "VX-max Img"=w6232, "Ypixels Img"=w6230, "Vy-min Img"=w6228, "Vy-max Img"=w6229, "Colormap"=w6234, "square pixels"=w6227, "square matrix"=w6226, "Angle Img"=w6225) -> (w6236:T12)
                    n3031 = call "2pparameters.vi"("Params in"=w6236, "command"="set") -> ()  [unwired: 1 out]
                    n3032 = local read "Vx-max draw"() -> (w6217:dbl)
                    n3033 = local read "Angle drawing"() -> (w6224:dbl)
                    n3034 = local read "Vx-min draw"() -> (w6218:dbl)
                    n3035 = local read "Vy-min draw"() -> (w6221:dbl)
                    n3036 = local read "ypixels draw"() -> (w6219:dbl)
                    n3037 = local read "Vy-max draw"() -> (w6220:dbl)
                    n3038 = local read "Square pixels"() -> (w6222:bool)
                    n3039 = local read "square matrix"() -> (w6223:bool)
                    n3040 = local read "xpixels draw"() -> (w6216:dbl)
                    n3041 = local read "Colormap"() -> (w6215:i32)
                    n3042 = call "2pparameters.vi"("command"="get") -> ("params out"=w6212:T12)  [unwired: 1 in]
                    n3043 = Bundle By Name(cluster=w6212, "Xpixels"=w6216, "Vxminref"=w6218, "Vxmaxref"=w6217, "Ypixels"=w6219, "Vyminref"=w6221, "Vymaxref"=w6220, "Colormap"=w6215, "square pixels"=w6222, "square matrix"=w6223, "Angle draw"=w6224) -> (w6213:T12)
                    n3044 = call "2pparameters.vi"("Params in"=w6213, "command"="set") -> ()  [unwired: 1 out]
                  }
                  frame #1 {
                    n3045 = Current VI's Path() -> (path=w6248:path)
                    n3046 = Strip Path(path=w6248) -> (stripped path=w6249:path)  [unwired: 1 out]
                    n3047 = Build Path(base path=w6249, name or relative path="subVIs\\Image\\SetROI_v3.vi") -> (appended path=w6247:path)
                    n3048 = call <vilib>:"Set Busy.vi"() -> ("error out"=w6245:errorcluster)  [unwired: 10 in, 1 out]
                    n3049 = Open VI Reference(type specifier VI Refnum (for type only)=refnum<vi> refnum, vi path=w6247, error in (no error)=w6245) -> (vi reference=w6243:refnum<vi>, error out=w6241:errorcluster)  [unwired: 3 in]
                    n3050 = call-by-ref "?"(reference=w6243, error in=w6241) -> (reference out=w6242:refnum<vi>, error out=w6240:errorcluster)  [unwired: 1 in]
                    n3051 = Close Reference(reference=w6242, error in (no error)=w6240) -> (error out=w6244:errorcluster)
                    n3052 = call <vilib>:"Unset Busy.vi"("error in (no error)"=w6244) -> ()  [unwired: 10 in, 1 out]
